vi "Recorder Encoder.vi"() -> ()   [LabVIEW 2011]
uses:
  <vilib>/Utility/file.llb/Write To Spreadsheet File (DBL).vi
panel:
  in  "Slide 2":dbl(slide) scale=-1000.0..1000.0
  in  "Slide":dbl(slide) scale=-1000.0..1000.0
  in  "File":bool
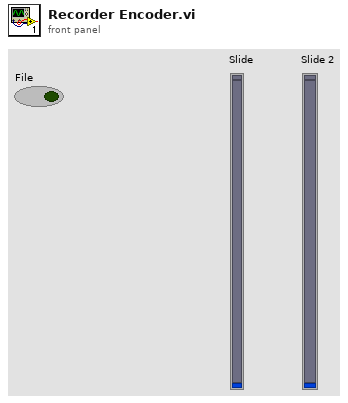
[diagram p1: front panel]
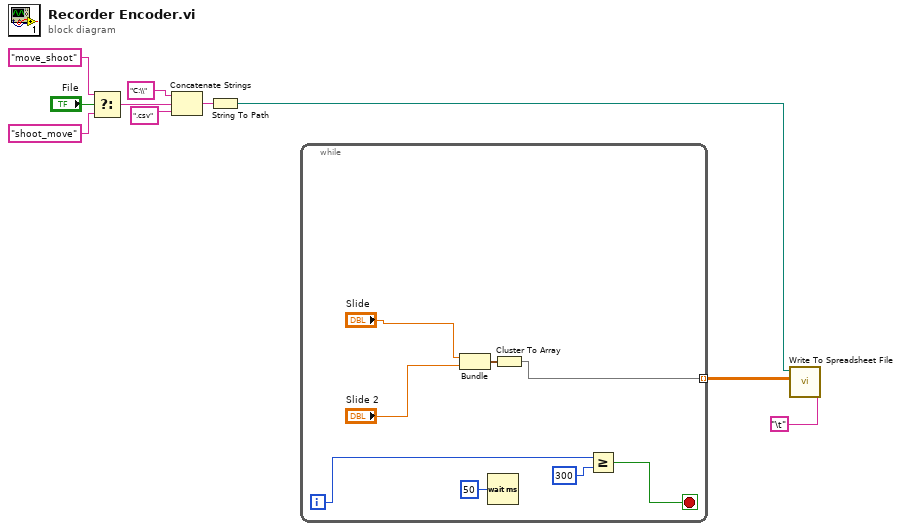
[diagram p0: block diagram]
diagram:
  n1 = Select(t="move_shoot", s="File", f="shoot_move") -> (s? t:f=w3:string)
  n2 = Concatenate Strings("C:\\", w3, ".csv") -> (w2:string)
  n3 = String To Path(string=w2) -> (path=w7:path)
  n4 = while {
    tunnel: [w11] -> w8 mode=indexing
    i -> [w17]
    stop <- w15 stop-if-true
    n5 = Bundle("Slide"="Slide", "Slide 2"="Slide 2") -> (w12:cluster{"Slide":dbl, "Slide 2":dbl})  [unwired: 1 in]
    n6 = Wait (ms)(milliseconds to wait=u32 50) -> ()  [unwired: 1 out]
    n7 = Cluster To Array(cluster=w12) -> (array=w11:dbl[])
    n8 = Greater Or Equal?(x=w17, y=300) -> (x >= y?=w15:bool)
  }
  n9 = call-poly <vilib>:"Write To Spreadsheet File.vi"("delimiter (\\t)"="\t", "2D data"=w8, "file path (dialog if empty)"=w7) -> ()  [unwired: 5 in, 1 out]
